vi "SetFormat.vi"(8 "Error In":errorcluster, 10 "Format Elements":T1[](array[typedef]), 11 "Keithley 6485 In":refnum<visa-resource-name>) -> (0 "Error Out":errorcluster, 3 "Keithley 6485 Out":refnum<visa-resource-name>)   [LabVIEW 2012, in "Keithley-6485.lvlib"]
uses:
  Keithley-6485.lvlib
  Controls/FormatElement.ctl
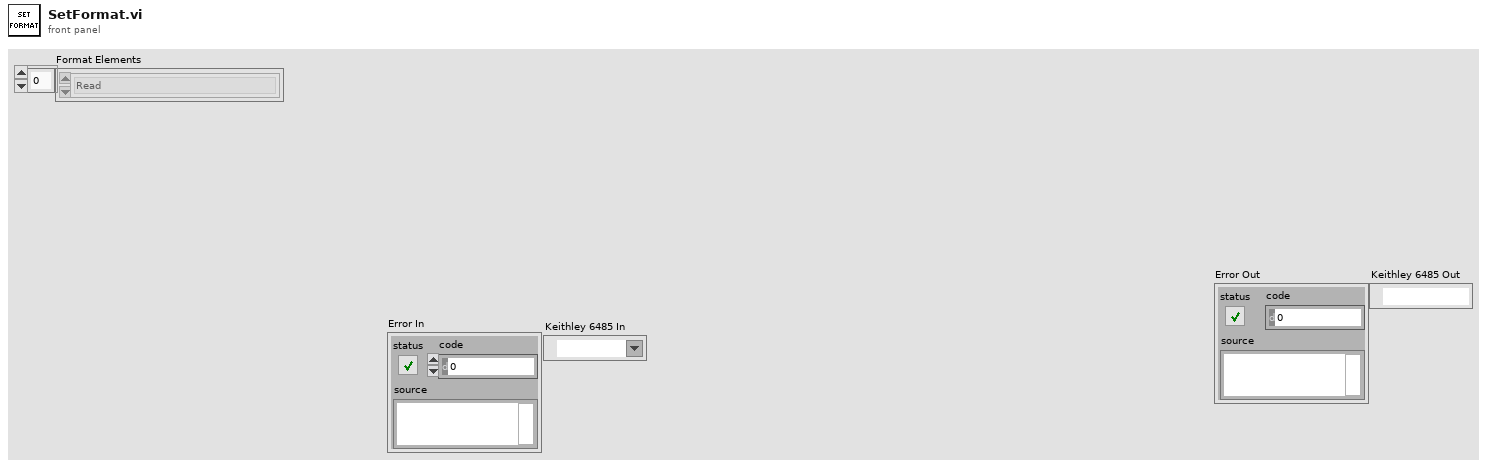
[diagram p1: front panel]
types:
  T1 = typedef "Keithley-6485.lvlib/FormatElement.ctl" = enum16{"Read", "Unit", "Time", "Status"}
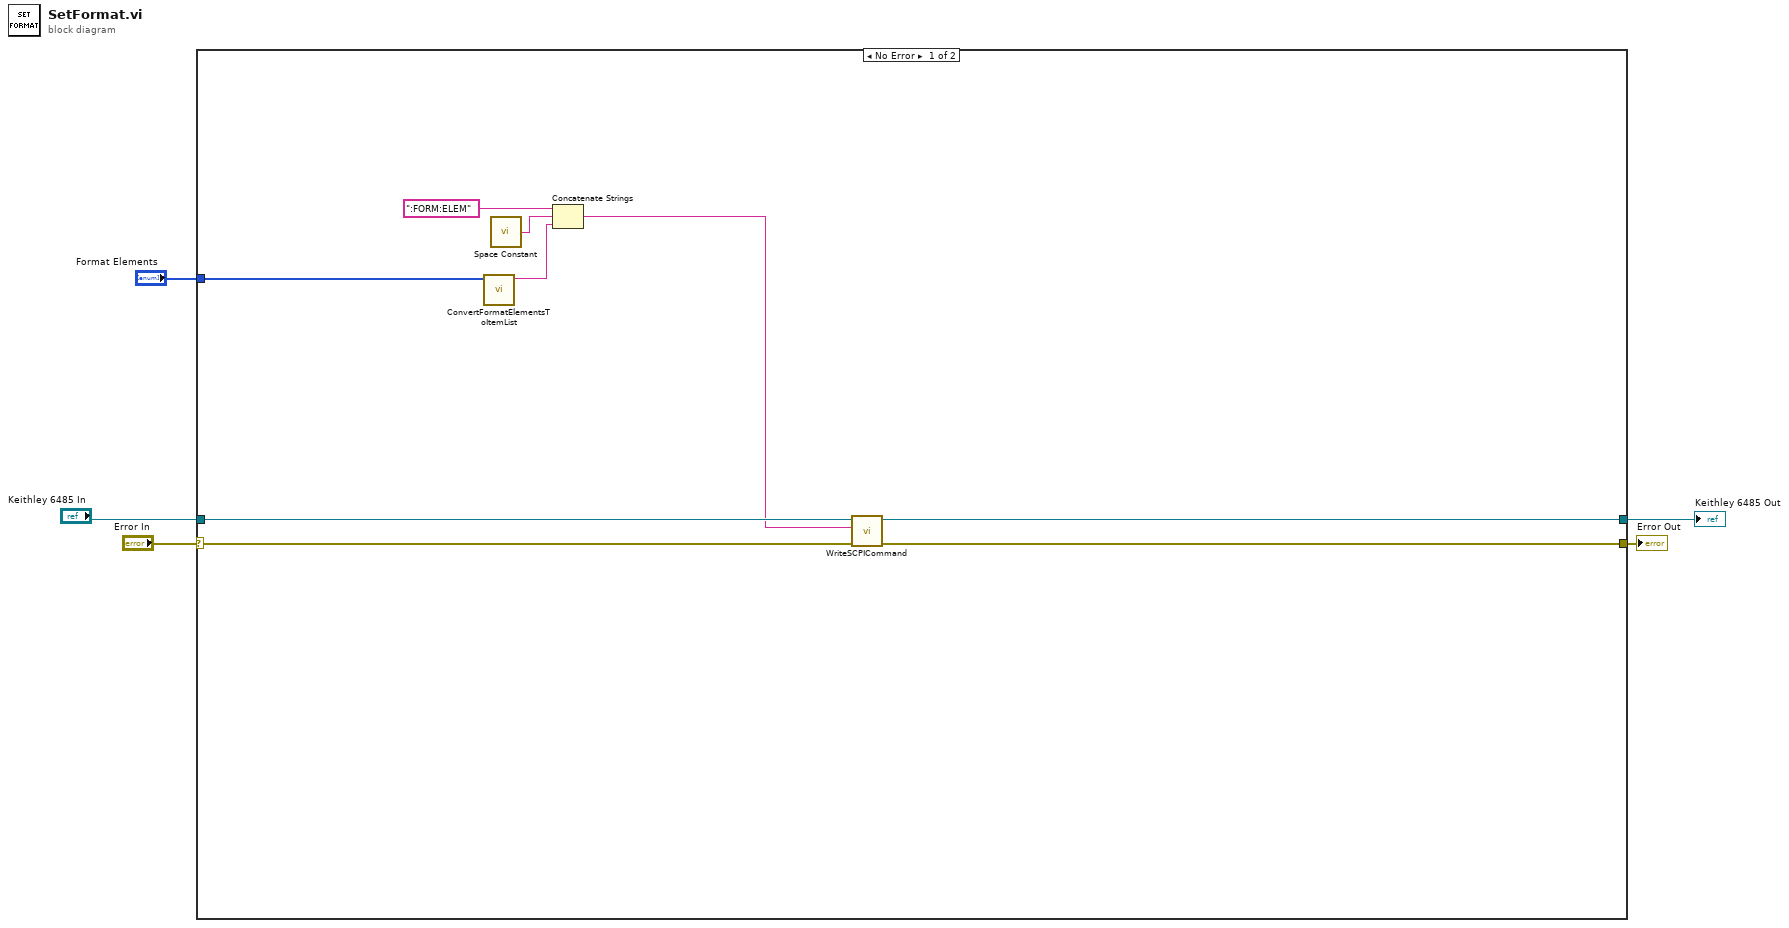
[diagram p0: block diagram]
diagram:
  n1 = case shown="No Error" "Error In" {
    selector: "Error In" -> [w14 w15]
    tunnel: [w13 w15] -> w4
    tunnel: [w12 w16] -> w3
    tunnel: "Keithley 6485 In" -> [w11 w16]
    tunnel: "Format Elements" -> [w6 _]
    frame No Error {
      n2 = call "ConvertFormatElementsToItemList.vi"("Format Elements"=w6) -> ("Item List"=w7:string)  [unwired: 10 in]
      n3 = call <vilib>:"Space Constant.vi"() -> ("String"=w9:string)
      n4 = Concatenate Strings(":FORM:ELEM", w9, w7) -> (w8:string)
      n5 = call "WriteSCPICommand.vi"("Error In"=w14, "SCPI Command"=w8, "Keithley 6482 In"=w11) -> ("Error Out"=w13:errorcluster, "Keithley 6482 Out"=w12:refnum<visa-resource-name>)  [unwired: 7 in]
    }
    frame Error {
    }
  }
  "Error Out" <- w4
  "Keithley 6485 Out" <- w3
